vi "Configure_E_Load.vi"(8 "error in (no error)":errorcluster, 9 "Function":T1, 10 "byte count":u32, 11 "VISA resource name in":refnum<visa-resource-name>) -> (0 "error out":errorcluster, 2 "Output":string, 3 "VISA resource name out":refnum<visa-resource-name>)   [LabVIEW 2025]
uses:
  BK Precision Function CTL.ctl
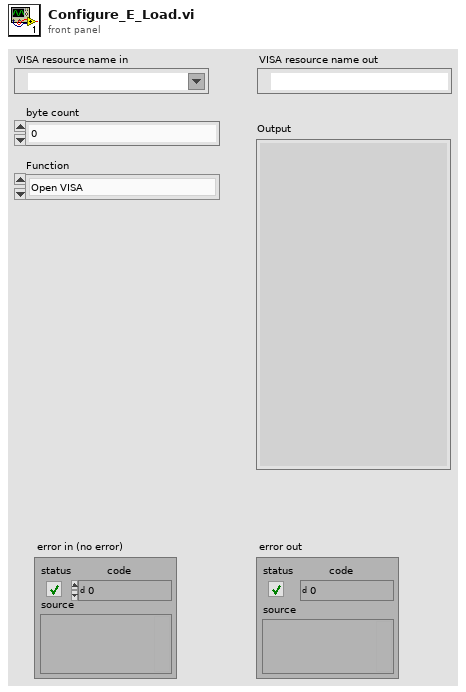
[diagram p1: front panel]
types:
  T1 = typedef "BK Precision Function CTL.ctl" = enum16{"Open VISA", "Close VISA", "Query IDN", "Set Voltage", "Set Current", "Measure Voltage", "Measure Current", "Enable/Disable Output"}
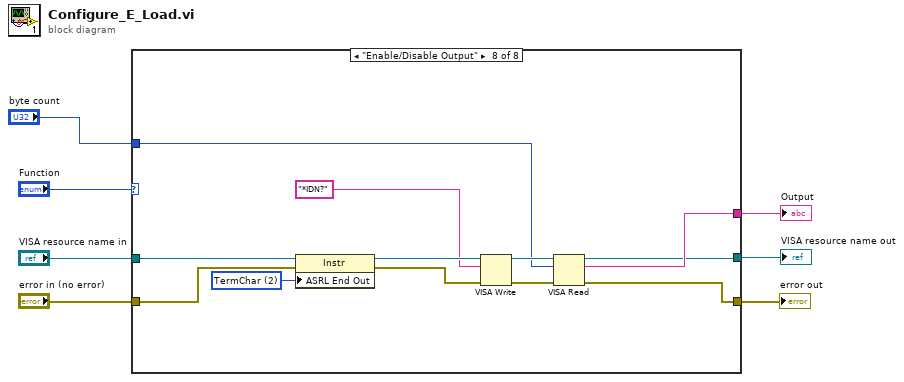
[diagram p0: block diagram]
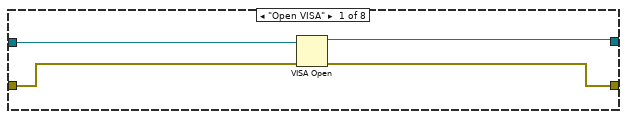
[diagram p2: hidden frame]
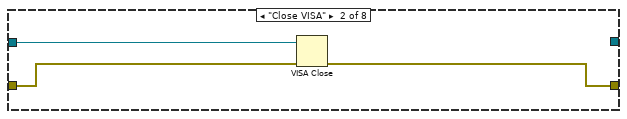
[diagram p3: hidden frame]
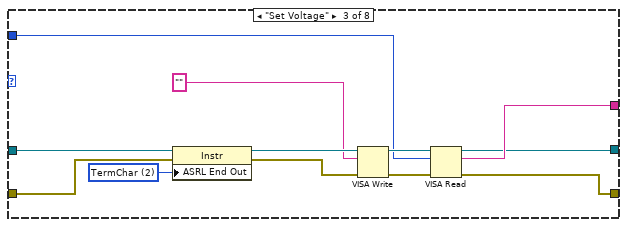
[diagram p4: hidden frame]
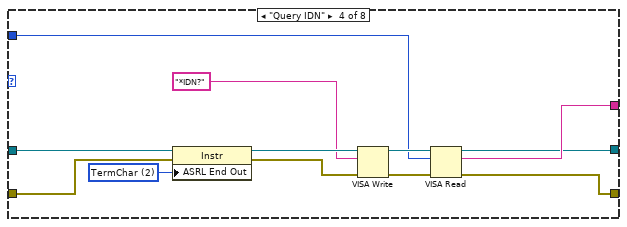
[diagram p5: hidden frame]
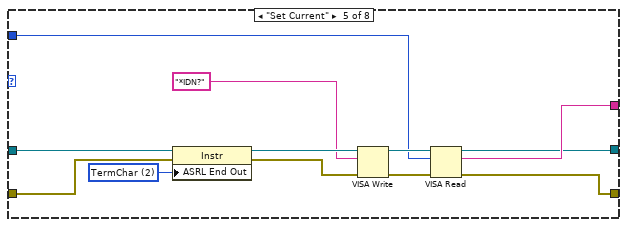
[diagram p6: hidden frame]
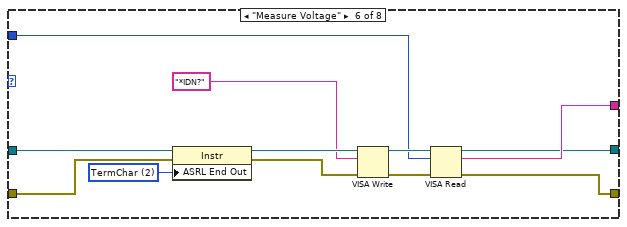
[diagram p7: hidden frame]
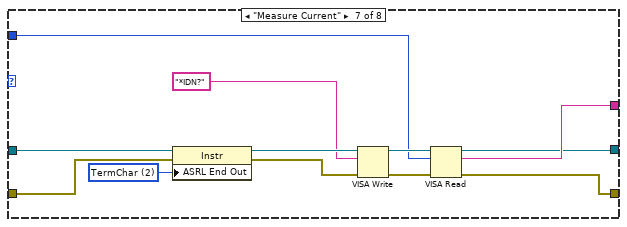
[diagram p8: hidden frame]
diagram:
  n1 = case shown="\"Enable/Disable Output\"" "Function" {
    tunnel: "VISA resource name in" -> [w11 w14 w26 w38 w50 w62 w74 w86]
    tunnel: [_ _ w22 w34 w46 w58 w70 w82] -> w6
    tunnel: [w10 _ w19 w31 w43 w55 w67 w79] -> w4
    tunnel: "error in (no error)" -> [w9 w13 w18 w30 w42 w54 w66 w78]
    tunnel: [w8 w12 w17 w29 w41 w53 w65 w77] -> w2
    tunnel: "byte count" -> [_ _ w15 w27 w39 w51 w63 w75]
    frame "Open VISA" {
      n2 = VISA Open(error in (no error)=w9, VISA resource name=w11) -> (VISA resource name=w10:refnum<visa-resource-name>, error out=w8:errorcluster)  [unwired: 3 in]
    }
    frame "Close VISA" {
      n3 = VISA Close(VISA resource name=w14, error in (no error)=w13) -> (error out=w12:errorcluster)
    }
    frame "Set Voltage" {
      w25 = u16 2 items=["None", "Last Bit", "TermChar", "Break"] ("Serial Settings:End Mode for Writes")
      n4 = property class="Instr"(reference=w26, error in=w18, "ASRL End Out"=w25) -> (reference out=w24:refnum<visa-resource-name>, error out=w23:errorcluster)
      n5 = VISA Write(VISA resource name=w24, write buffer="", error in (no error)=w23) -> (VISA resource name out=w21:refnum<visa-resource-name>, error out=w20:errorcluster)  [unwired: 1 out]
      n6 = VISA Read(VISA resource name=w21, byte count=w15, error in (no error)=w20) -> (VISA resource name out=w19:refnum<visa-resource-name>, read buffer=w22:string, error out=w17:errorcluster)  [unwired: 1 out]
    }
    frame "Query IDN" {
      w37 = u16 2 items=["None", "Last Bit", "TermChar", "Break"] ("Serial Settings:End Mode for Writes")
      n7 = property class="Instr"(reference=w38, error in=w30, "ASRL End Out"=w37) -> (reference out=w36:refnum<visa-resource-name>, error out=w35:errorcluster)
      n8 = VISA Write(VISA resource name=w36, write buffer="*IDN?", error in (no error)=w35) -> (VISA resource name out=w33:refnum<visa-resource-name>, error out=w32:errorcluster)  [unwired: 1 out]
      n9 = VISA Read(VISA resource name=w33, byte count=w27, error in (no error)=w32) -> (VISA resource name out=w31:refnum<visa-resource-name>, read buffer=w34:string, error out=w29:errorcluster)  [unwired: 1 out]
    }
    frame "Set Current" {
      w49 = u16 2 items=["None", "Last Bit", "TermChar", "Break"] ("Serial Settings:End Mode for Writes")
      n10 = property class="Instr"(reference=w50, error in=w42, "ASRL End Out"=w49) -> (reference out=w48:refnum<visa-resource-name>, error out=w47:errorcluster)
      n11 = VISA Write(VISA resource name=w48, write buffer="*IDN?", error in (no error)=w47) -> (VISA resource name out=w45:refnum<visa-resource-name>, error out=w44:errorcluster)  [unwired: 1 out]
      n12 = VISA Read(VISA resource name=w45, byte count=w39, error in (no error)=w44) -> (VISA resource name out=w43:refnum<visa-resource-name>, read buffer=w46:string, error out=w41:errorcluster)  [unwired: 1 out]
    }
    frame "Measure Voltage" {
      w61 = u16 2 items=["None", "Last Bit", "TermChar", "Break"] ("Serial Settings:End Mode for Writes")
      n13 = property class="Instr"(reference=w62, error in=w54, "ASRL End Out"=w61) -> (reference out=w60:refnum<visa-resource-name>, error out=w59:errorcluster)
      n14 = VISA Write(VISA resource name=w60, write buffer="*IDN?", error in (no error)=w59) -> (VISA resource name out=w57:refnum<visa-resource-name>, error out=w56:errorcluster)  [unwired: 1 out]
      n15 = VISA Read(VISA resource name=w57, byte count=w51, error in (no error)=w56) -> (VISA resource name out=w55:refnum<visa-resource-name>, read buffer=w58:string, error out=w53:errorcluster)  [unwired: 1 out]
    }
    frame "Measure Current" {
      w73 = u16 2 items=["None", "Last Bit", "TermChar", "Break"] ("Serial Settings:End Mode for Writes")
      n16 = property class="Instr"(reference=w74, error in=w66, "ASRL End Out"=w73) -> (reference out=w72:refnum<visa-resource-name>, error out=w71:errorcluster)
      n17 = VISA Write(VISA resource name=w72, write buffer="*IDN?", error in (no error)=w71) -> (VISA resource name out=w69:refnum<visa-resource-name>, error out=w68:errorcluster)  [unwired: 1 out]
      n18 = VISA Read(VISA resource name=w69, byte count=w63, error in (no error)=w68) -> (VISA resource name out=w67:refnum<visa-resource-name>, read buffer=w70:string, error out=w65:errorcluster)  [unwired: 1 out]
    }
    frame "Enable/Disable Output" {
      w85 = u16 2 items=["None", "Last Bit", "TermChar", "Break"] ("Serial Settings:End Mode for Writes")
      n19 = property class="Instr"(reference=w86, error in=w78, "ASRL End Out"=w85) -> (reference out=w84:refnum<visa-resource-name>, error out=w83:errorcluster)
      n20 = VISA Write(VISA resource name=w84, write buffer="*IDN?", error in (no error)=w83) -> (VISA resource name out=w81:refnum<visa-resource-name>, error out=w80:errorcluster)  [unwired: 1 out]
      n21 = VISA Read(VISA resource name=w81, byte count=w75, error in (no error)=w80) -> (VISA resource name out=w79:refnum<visa-resource-name>, read buffer=w82:string, error out=w77:errorcluster)  [unwired: 1 out]
    }
  }
  "Output" <- w6
  "VISA resource name out" <- w4
  "error out" <- w2
